vi "Example Graph - Position Callback.vi"(4 "Position":refnum<user-event>, 5 "Event Data":cluster{"sender":refnum<k24>, "x":i16, "y":i16}, 6 "Control Ref":refnum<k24>, 7 "Event Common Data":T1) -> ()   [LabVIEW 2010]
uses:
  C:/tf/play/labview/Tinkerforge.dll
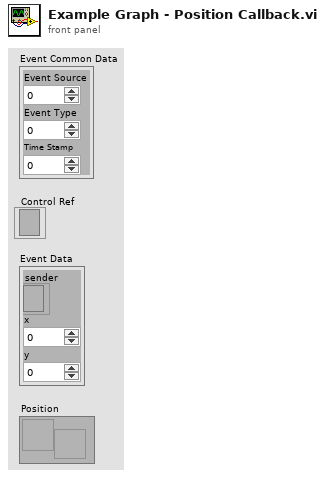
[diagram p1: front panel]
types:
  T1 = cluster{"Event Source":i32, "Event Type":u32, "Time Stamp":u32}
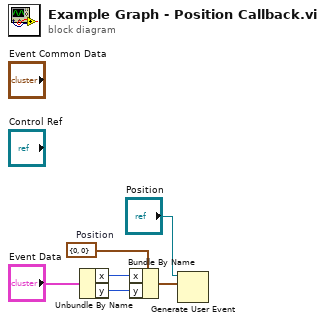
[diagram p0: block diagram]
diagram:
  w3 = cluster{"x":i16, "y":i16} {"x"=0, "y"=0}  # Position
  n1 = Unbundle By Name("Event Data") -> ("x"=w5:i16, "y"=w4:i16)
  n2 = Bundle By Name(cluster=w3, "x"=w5, "y"=w4) -> (w2:cluster{"x":i16, "y":i16})
  n3 = Generate User Event(user event="Position", event data cluster=w2) -> ()  [unwired: 1 in, 2 out]
